vi "Save Image To File.vi"   [LabVIEW 2020, in "G-Image.lvlib"]
doc: "<b>This VI is polymorphic.</b>\n\nSaves an image in the selected format to disk.\n\n<b>Path In</b> can be a standard path type, or a UTF-8 encoded string."
uses:
  G-Image.lvlib
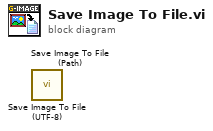
[diagram p0: block diagram]
diagram:
  n1 = call "Save Image To File (UTF-8).vi"() -> ()  [unwired: 10 in, 2 out]
  n2 = call "Save Image To File (Path).vi"() -> ()  [unwired: 10 in, 2 out]
